vi "Set SysDef Configuration.vi"(8 "error in (no error)":errorcluster, 10 "Configuration":T2={"Name"="", "Description"="", "Protocol"="", "RS232 Config"={"Port"="COM1", "Baud Rate"=9600, "Data Bits"=8, "Parity"=enum."None", "Stop Bits"=10, "Flow Control"=0, "XON"=enum."DC1", "XOFF"=enum."DC3", "End Read on Termination Character"=TRUE, "End Write on Termination Character"=TRUE, "Termination Character"=10}, "MetaData Globals"=[], "Message Groups"=[], "GPIB Config"={"VISA Resource"="GPIB0::2::INSTR", "Enable Termination Character"=TRUE, "Termination Character"=10, "Timeout"=2000, "Append Write Termination Character"=FALSE}, "TCPIP Config"={"IP Address"="localhost", "Port"=0}, "Decimation"=0, "UDP Config"={"Local IP Address"="localhost", "Local Port"=8888, "Target IP Address"="localhost", "Target Port"=8888}} {"GPIB Config"."Termination Character" format="%.0x"; "RS232 Config"."Termination Character" format="%.0x"; "RS232 Config"."Flow Control" items=["None"=0, "XON/XOFF"=1, "RTS/CTS"=2, "DTR/DSR"=4]; "RS232 Config"."Stop Bits" items=["1.0"=10, "1.5"=15, "2.0"=20]; "RS232 Config"."Data Bits" min=5 max=8 step=1; "RS232 Config"."Baud Rate" items=["75"=75, "110"=110, "134"=134, "150"=150, "300"=300, "600"=600, "1200"=1200, "1800"=1800, "2400"=2400, "4800"=4800, "7200"=7200, "9600"=9600, "14400"=14400, "19200"=19200, "28800"=28800, "38400"=38400, "56000"=56000, "57600"=57600, "115200"=115200, "128000"=128000, "230400"=230400, "460800"=460800, "921600"=921600, "1843200"=1843200, "3000000"=3000000]}, 11 "Node Ptr":u64 format="%.0x") -> (0 "error out":errorcluster, 3 "Ref out":T1=18446744073709551615 format="%.0x")   [LabVIEW 2019, in "Instrument Addon System Explorer.lvlib"]
uses:
  Instrument Addon System Explorer.lvlib
  Instrument Custom Device SysDef Configuration V1.0.1.ctl
  Shared/Types/RSXXX Port Settings.ctl
  MetaData Channel Configuration.ctl
  Shared/Types/MetaData Parameters.ctl
  Shared/Types/Protocol Data Type.ctl
  Shared/Types/Metadata Channel Type.ctl
  Shared/Types/Type Cast Type.ctl
  Shared/Types/Endian.ctl
  Types/Channel Properties.ctl
  Message Group Configuration.ctl
  Message Configuration.ctl
  Command Message Configuration.ctl
  Shared/Types/Command Parameters.ctl
  Shared/Types/Linked Channel Cluster.ctl
  Response Message Configuration.ctl
  Shared/Types/Response Parameters.ctl
  Shared/Types/Response Wait Type.ctl
  Data Channel Configuration.ctl
  Shared/Types/Data Parameters.ctl
  Shared/Types/Data Channel Type.ctl
  Shared/Types/Message Parameters.ctl
  Shared/Types/Message Generation Type.ctl
  Shared/Types/Trigger Parameters.ctl
  Shared/Types/VISA Settings.ctl
  Shared/Types/TCPIP Settings.ctl
  Shared/Types/UDP Settings.ctl
  <vilib>/NI VeriStand/Custom Device API/Custom Device Item Ref.ctl
  Shared/Types/FG Control.ctl
  <vilib>/NI VeriStand/Custom Device API/Custom Device Channel.ctl
  <vilib>/NI VeriStand/Custom Device API/Custom Device Channel Type.ctl
  Shared/Constants.vi
  <vilib>/NI VeriStand/Custom Device API/NI VeriStand - Get Item Property.vi
  <vilib>/NI VeriStand/Custom Device API/Get Item Property (U32).vi
  <vilib>/NI VeriStand/Custom Device API/Set Item Property (U32).vi
  <vilib>/NI VeriStand/Custom Device API/Get Item Property (String).vi
  <vilib>/NI VeriStand/Custom Device API/Set Item Property (String).vi
  <vilib>/NI VeriStand/Custom Device API/Get Item Property (Boolean).vi
  <vilib>/NI VeriStand/Custom Device API/Set Item Property (Boolean).vi
  <vilib>/NI VeriStand/Custom Device API/Get Item Property (String Array).vi
  <vilib>/NI VeriStand/Custom Device API/Set Item Property (String Array).vi
  <vilib>/NI VeriStand/Custom Device API/NI VeriStand - Get Item Children.vi
  <vilib>/NI VeriStand/Custom Device API/NI VeriStand - Set Custom Device Channel Value Table.vi
  <vilib>/NI VeriStand/Custom Device API/Get Item Property (Double).vi
  <vilib>/NI VeriStand/Custom Device API/Set Item Property (Double).vi
  <vilib>/NI VeriStand/Custom Device API/Custom Device API.lvlib
  Shared/Instrument Addon Shared.lvlib
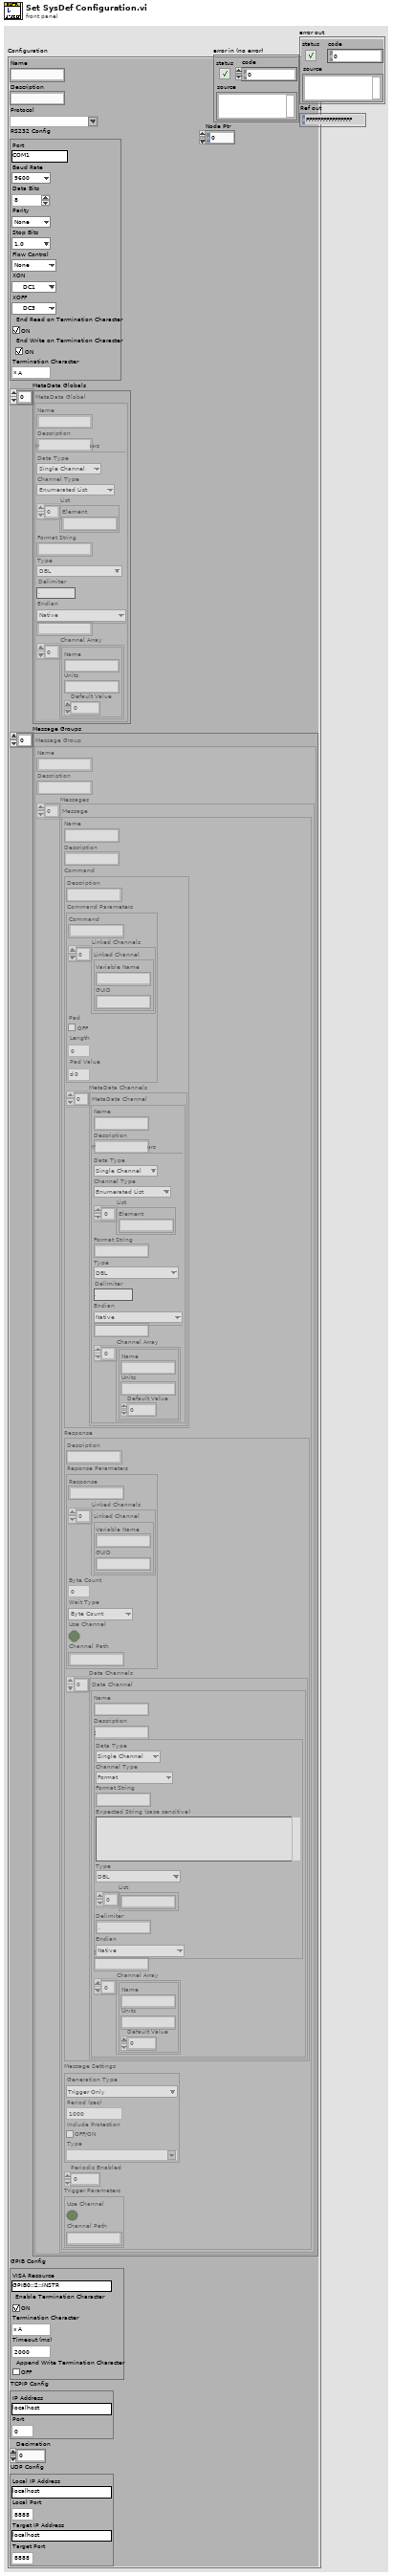
[diagram p1: front panel]
types:
  T1 = typedef "Custom Device API.lvlib/Custom Device Item Ref.ctl" = u64
  T2 = typedef "Instrument Addon System Explorer.lvlib/Instrument Custom Device SysDef Configuration V1.0.1.ctl" = cluster{"Name":string, "Description":string, "Protocol":string, "RS232 Config":T3, "MetaData Globals":T4[], "Message Groups":T11[], "GPIB Config":T25, "TCPIP Config":T26, "Decimation":u32, "UDP Config":T27}
  T3 = typedef "Instrument Addon Shared.lvlib/RSXXX Port Settings.ctl" = cluster{"Port":string, "Baud Rate":u32, "Data Bits":u16, "Parity":enum16{"None", "Odd", "Even", "Mark", "Space"}, "Stop Bits":u16, "Flow Control":u16, "XON":enum16{"NUL", "SOH", "STX", "ETX", "EOT", "ENQ", "ACK", "BEL", "BS", "HT", "LF", "VT", "FF", "CR", "SO", "SI", "DLE", "DC1", "DC2", "DC3", "DC4", "NAK", "SYN", "ETB", "CAN", "EM", "SUB", "ESC", "FS", "GS", "RS", "US", "SP", "!", "\"", "#", "$", "%", "&", "'", "(", ")", "*", "+", ",", "- (-)", ".", "/", "0", "1", "2", "3", "4", "5", "6", "7", "8", "9", ":", ";", "<", "=", ">", "?", "@", "A", "B", "C", "D", "E", "F", "G", "H", "I", "J", "K", "L", "M", "N", "O", "P", "Q", "R", "S", "T", "U", "V", "W", "X", "Y", "Z", "[", "\\", "]", "^", "_", "`", "a", "b", "c", "d", "e", "f", "g", "h", "i", "j", "k", "l", "m", "n", "o", "p", "q", "r", "s", "t", "u", "v", "w", "x", "y", "z", "{", "|", "}", "~"}, "XOFF":enum16{"NUL", "SOH", "STX", "ETX", "EOT", "ENQ", "ACK", "BEL", "BS", "HT", "LF", "VT", "FF", "CR", "SO", "SI", "DLE", "DC1", "DC2", "DC3", "DC4", "NAK", "SYN", "ETB", "CAN", "EM", "SUB", "ESC", "FS", "GS", "RS", "US", "SP", "!", "\"", "#", "$", "%", "&", "'", "(", ")", "*", "+", ",", "- (-)", ".", "/", "0", "1", "2", "3", "4", "5", "6", "7", "8", "9", ":", ";", "<", "=", ">", "?", "@", "A", "B", "C", "D", "E", "F", "G", "H", "I", "J", "K", "L", "M", "N", "O", "P", "Q", "R", "S", "T", "U", "V", "W", "X", "Y", "Z", "[", "\\", "]", "^", "_", "`", "a", "b", "c", "d", "e", "f", "g", "h", "i", "j", "k", "l", "m", "n", "o", "p", "q", "r", "s", "t", "u", "v", "w", "x", "y", "z", "{", "|", "}", "~"}, "End Read on Termination Character":bool, "End Write on Termination Character":bool, "Termination Character":u8}
  T4 = typedef "Instrument Addon System Explorer.lvlib/MetaData Channel Configuration.ctl" = cluster{"Name":string, "Description":string, "MetaData Parameters":T5, "Config GUID":string, "Channel Array":T10[]}
  T5 = typedef "Instrument Addon Shared.lvlib/MetaData Parameters.ctl" = cluster{"Data Type":T6, "Channel Type":T7, "List":string[], "Format String":string, "Type":T8, "Delimiter":string, "Endian":T9}
  T6 = typedef "Instrument Addon Shared.lvlib/Protocol Data Type.ctl" = enum16{"Single Channel", "Array"}
  T7 = typedef "Instrument Addon Shared.lvlib/Metadata Channel Type.ctl" = enum16{"Enumerated List", "Format", "Type Cast"}
  T8 = typedef "Instrument Addon Shared.lvlib/Type Cast Type.ctl" = enum16{"DBL", "SGL", "U64", "U32", "U16", "U8", "I64", "I32", "I16", "I8"}
  T9 = typedef "Instrument Addon Shared.lvlib/Endian.ctl" = enum16{"Native", "Little", "Big"}
  T10 = typedef "Instrument Addon System Explorer.lvlib/Channel Properties.ctl" = cluster{"Name":string, "Units":string, "Default Value":dbl}
  T11 = typedef "Instrument Addon System Explorer.lvlib/Message Group Configuration.ctl" = cluster{"Name":string, "Description":string, "Messages":T12[]}
  T12 = typedef "Instrument Addon System Explorer.lvlib/Message Configuration.ctl" = cluster{"Name":string, "Description":string, "Command":T13, "Response":T16, "Message Settings":T22, "Periodic Enabled":dbl, "Trigger Parameters":T24}
  T13 = typedef "Instrument Addon System Explorer.lvlib/Command Message Configuration.ctl" = cluster{"Description":string, "Command Parameters":T14, "MetaData Channels":T4[]}
  T14 = typedef "Instrument Addon Shared.lvlib/Command Parameters.ctl" = cluster{"Command":string, "Linked Channels":T15[], "Pad":bool, "Length":u32, "Pad Value":u8}
  T15 = typedef "Instrument Addon Shared.lvlib/Linked Channel Cluster.ctl" = cluster{"Variable Name":string, "GUID":string}
  T16 = typedef "Instrument Addon System Explorer.lvlib/Response Message Configuration.ctl" = cluster{"Description":string, "Reponse Parameters":T17, "Data Channels":T19[]}
  T17 = typedef "Instrument Addon Shared.lvlib/Response Parameters.ctl" = cluster{"Response":string, "Linked Channels":T15[], "Type Value":dbl, "Wait Type":T18, "Use Channel":bool, "Channel Path":string}
  T18 = typedef "Instrument Addon Shared.lvlib/Response Wait Type.ctl" = enum16{"Byte Count", "Wait sec"}
  T19 = typedef "Instrument Addon System Explorer.lvlib/Data Channel Configuration.ctl" = cluster{"Name":string, "Description":string, "Data Parameters":T20, "Config GUID":string, "Channel Array":T10[]}
  T20 = typedef "Instrument Addon Shared.lvlib/Data Parameters.ctl" = cluster{"Data Type":T6, "Channel Type":T21, "Format String":string, "Expected String":string, "Type":T8, "List":string[], "Delimiter":string, "Endian":T9}
  T21 = typedef "Instrument Addon Shared.lvlib/Data Channel Type.ctl" = enum16{"Format", "Comparison", "Type Cast", "Enumerated List"}
  T22 = typedef "Instrument Addon Shared.lvlib/Message Parameters.ctl" = cluster{"Generation Type":T23, "Period":dbl, "Include Protection":bool, "Type":string}
  T23 = typedef "Instrument Addon Shared.lvlib/Message Generation Type.ctl" = enum16{"Trigger Only", "Periodic & Trigger", "Value Change & Trigger"}
  T24 = typedef "Instrument Addon Shared.lvlib/Trigger Parameters.ctl" = cluster{"Use Channel":bool, "Channel Path":string}
  T25 = typedef "Instrument Addon Shared.lvlib/VISA Settings.ctl" = cluster{"VISA Resource":string, "Enable Termination Character":bool, "Termination Character":u8, "Timeout":u32, "Append Write Termination Character":bool}
  T26 = typedef "Instrument Addon Shared.lvlib/TCPIP Settings.ctl" = cluster{"IP Address":string, "Port":u16}
  T27 = typedef "Instrument Addon Shared.lvlib/UDP Settings.ctl" = cluster{"Local IP Address":string, "Local Port":u16, "Target IP Address":string, "Target Port":u16}
  T28 = typedef "Instrument Addon Shared.lvlib/FG Control.ctl" = enum16{"Get", "Set"}
  T29 = typedef "Custom Device API.lvlib/Custom Device Channel.ctl" = cluster{"Type":T30, "Units":string, "Default Value":dbl, "Faultable":bool, "Scalable":bool}
  T30 = typedef "Custom Device API.lvlib/Custom Device Channel Type.ctl" = enum16{"Input", "Output"}
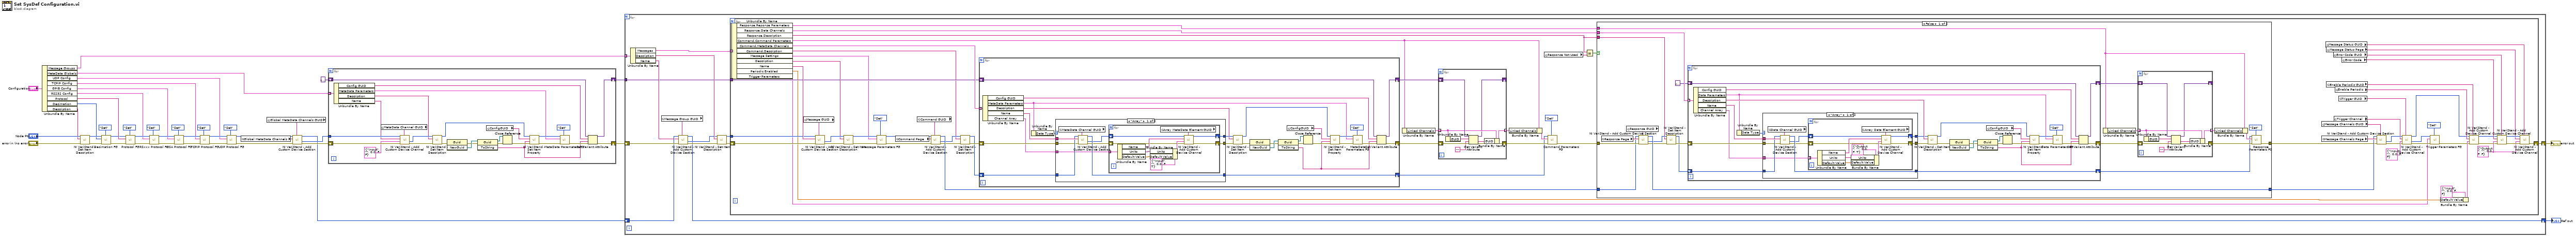
[diagram p0: block diagram]
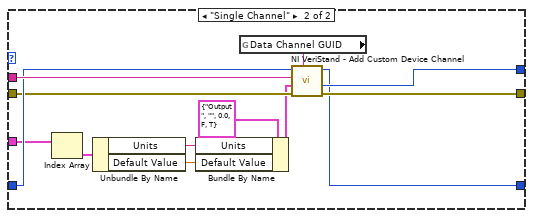
[diagram p2: hidden frame]
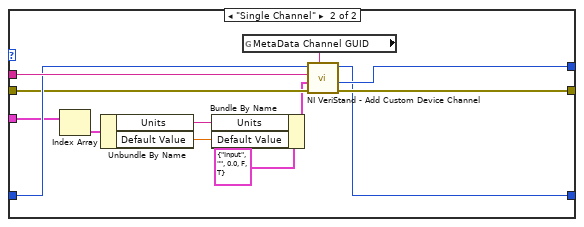
[diagram p4: hidden frame]
diagram:
  n1 = Unbundle By Name("Configuration") -> ("Message Groups"=w24:T11[], "MetaData Globals"=w29:T4[], "UDP Config"=w1:T27, "TCPIP Config"=w13:T26, "GPIB Config"=w16:T25, "RS232 Config"=w32:T3, "Protocol"=w33:string, "Decimation"=w7:u32, "Description"=w34:string)
  n2 = call <vilib>:"NI VeriStand - Set Item Description.vi"("error in (no error)"="error in (no error)", "Description"=w34, "Item Ref in"="Node Ptr") -> ("error out"=w10:errorcluster, "Item Ref out"=w35:T1)  [unwired: 6 in, 1 out]
  n3 = call "Decimation FG.vi"("Action"=FG_Control."Set", "error in (no error)"=w10, "Decimation"=w7, "Device Item Ref in"=w35) -> ("error out"=w9:errorcluster, "Item Ref out"=w11:T1)  [unwired: 5 in, 1 out]
  n4 = call "Protocol FG.vi"("Action"=FG_Control."Set", "error in (no error)"=w9, "Protocol"=w33, "Device Item Ref in"=w11) -> ("error out"=w41:errorcluster, "Item Ref out"=w40:T1)  [unwired: 5 in, 1 out]
  n5 = call "RSxxx Protocol FG.vi"("Action"=FG_Control."Set", "error in (no error)"=w41, "Serial Config"=w32, "Device Item Ref in"=w40) -> ("error out"=w19:errorcluster, "Item Ref out"=w17:T1)  [unwired: 5 in, 1 out]
  n6 = call "VISA Protocol FG.vi"("Action"=FG_Control."Set", "error in (no error)"=w19, "VISA Config"=w16, "Device Item Ref in"=w17) -> ("error out"=w18:errorcluster, "Item Ref out"=w14:T1)  [unwired: 5 in, 1 out]
  n7 = call "TCPIP Protocol FG.vi"("Action"=FG_Control."Set", "error in (no error)"=w18, "TCP/IP Config"=w13, "Device Item Ref in"=w14) -> ("error out"=w6:errorcluster, "Item Ref out"=w4:T1)  [unwired: 5 in, 1 out]
  n8 = call "UDP Protocol FG.vi"("Action"=FG_Control."Set", "error in (no error)"=w6, "UDP Config"=w1, "Device Item Ref in"=w4) -> ("error out"=w5:errorcluster, "Item Ref out"=w3:T1)  [unwired: 5 in, 1 out]
  n9 = global read "Constants.vi" "Global MetaData Channels"() -> (w30:string)
  n10 = global read "Constants.vi" "Global MetaData Channels GUID"() -> (w31:string)
  n11 = call <vilib>:"NI VeriStand - Add Custom Device Section.vi"("GUID (Default Section)"=w31, "error in (no error)"=w5, "Section Name"=w30, "Parent Ref in"=w3) -> ("error out"=w28:errorcluster, "Section Ptr"=w27:T1, "Parent Ref out"=w23:T1)  [unwired: 4 in, 1 out]
  n12 = for {
    tunnel: w29 -> [w69] mode=indexing
    tunnel: w27 -> [w61]
    shift-right: [w45] -> w22
    shift-left: variant ("variant") -> [w46]
    shift-right: [w44] -> w25
    shift-left: w28 -> [w62]
    n13 = Unbundle By Name(w69) -> ("Config GUID"=w48:string, "MetaData Parameters"=w50:T5, "Description"=w54:string, "Name"=w59:string)
    n14 = global read "Constants.vi" "MetaData Channel GUID"() -> (w60:string)
    n15 = call <vilib>:"NI VeriStand - Add Custom Device Channel.vi"("GUID (Default Channel)"=w60, "error in (no error)"=w62, "Channel"=T29 {"Type"=enum."Input", "Units"="", "Default Value"=0.0, "Faultable"=FALSE, "Scalable"=FALSE}, "Channel Name"=w59, "Parent Ref in"=w61) -> ("error out"=w58:errorcluster, "Channel Ref"=w56:T1)  [unwired: 3 in, 2 out]
    n16 = call <vilib>:"NI VeriStand - Set Item Description.vi"("error in (no error)"=w58, "Description"=w54, "Item Ref in"=w56) -> ("error out"=w57:errorcluster, "Item Ref out"=w55:T1)  [unwired: 6 in, 1 out]
    n17 = invoke class="Guid" method="NewGuid"(error in=w57) -> (error out=w65:errorcluster, "NewGuid"=w66:refnum<k24>)  [unwired: 2 in, 1 out]
    n18 = invoke class="Guid" method="ToString"(reference=w66, error in=w65) -> (reference out=w67:refnum<k24>, error out=w64:errorcluster, "ToString"=w47:string)  [unwired: 1 in]
    n19 = global read "Constants.vi" "ConfigGUID"() -> (w68:string)
    n20 = Close Reference(reference=w67, error in (no error)=w64) -> (error out=w63:errorcluster)
    n21 = call-poly <vilib>:"NI VeriStand - Set Item Property.vi"("error in (no error)"=w63, "Value"=w47, "Property Name"=w68, "Item Ref in"=w55) -> ("error out"=w53:errorcluster, "Item Ref out"=w52:T1)  [unwired: 5 in, 1 out]
    n22 = call "MetaData Parameters FG.vi"("Action"=FG_Control."Set", "error in (no error)"=w53, "MetaData Parameters"=w50, "Item Ref in"=w52) -> ("error out"=w49:errorcluster)  [unwired: 5 in, 2 out]
    n23 = Set Variant Attribute(Variant=w46, name=w48, value=w47, error in=w49) -> (Variant out=w45:variant, error out=w44:errorcluster)  [unwired: 1 out]
  }
  n24 = for {
    shift-right: [w72] -> w21
    shift-left: w25 -> [w82]
    tunnel: w24 -> [w81] mode=indexing
    tunnel: w22 -> [w73]
    shift-right: [w70] -> w20
    shift-left: w23 -> [w79]
    n25 = Unbundle By Name(w81) -> ("Messages"=w76:T12[], "Description"=w77:string, "Name"=w78:string)
    n26 = global read "Constants.vi" "Message Group GUID"() -> (w83:string)
    n27 = call <vilib>:"NI VeriStand - Add Custom Device Section.vi"("GUID (Default Section)"=w83, "error in (no error)"=w82, "Section Name"=w78, "Parent Ref in"=w79) -> ("error out"=w80:errorcluster, "Section Ptr"=w71:T1, "Parent Ref out"=w70:T1)  [unwired: 4 in, 1 out]
    n28 = call <vilib>:"NI VeriStand - Set Item Description.vi"("error in (no error)"=w80, "Description"=w77, "Item Ref in"=w71) -> ("error out"=w75:errorcluster, "Item Ref out"=w74:T1)  [unwired: 6 in, 1 out]
    n29 = for {
      tunnel: w76 -> [w152] mode=indexing
      shift-right: [w110] -> w72
      shift-left: w75 -> [w132]
      tunnel: w74 -> [w133]
      tunnel: w73 -> [w113]
      w137 = T29 {"Type"=enum."Output", "Units"="", "Default Value"=0.0, "Faultable"=FALSE, "Scalable"=FALSE} ("Channel")
      n30 = Unbundle By Name(w152) -> ("Response.Reponse Parameters"=w111:T17, "Response.Data Channels"=w114:T19[], "Response.Description"=w92:string, "Command.Command Parameters"=w121:T14, "Command.MetaData Channels"=w126:T4[], "Command.Description"=w105:string, "Message Settings"=w98:T22, "Description"=w128:string, "Name"=w134:string, "Periodic Enabled"=w90:dbl, "Trigger Parameters"=w84:T24)
      n31 = global read "Constants.vi" "Message GUID"() -> (w150:string)
      n32 = call <vilib>:"NI VeriStand - Add Custom Device Section.vi"("GUID (Default Section)"=w150, "error in (no error)"=w132, "Section Name"=w134, "Parent Ref in"=w133) -> ("error out"=w131:errorcluster, "Section Ptr"=w129:T1)  [unwired: 4 in, 2 out]
      n33 = call <vilib>:"NI VeriStand - Set Item Description.vi"("error in (no error)"=w131, "Description"=w128, "Item Ref in"=w129) -> ("error out"=w130:errorcluster, "Item Ref out"=w103:T1)  [unwired: 6 in, 1 out]
      n34 = call "Message Parameters FG.vi"("Action"=FG_Control."Set", "error in (no error)"=w130, "Message Settings"=w98, "Item Ref in"=w103) -> ("error out"=w104:errorcluster, "Item Ref out"=w102:T1)  [unwired: 5 in, 1 out]
      n35 = global read "Constants.vi" "Command Page"() -> (w140:string)
      n36 = global read "Constants.vi" "Command GUID"() -> (w141:string)
      n37 = call <vilib>:"NI VeriStand - Add Custom Device Section.vi"("GUID (Default Section)"=w141, "error in (no error)"=w104, "Section Name"=w140, "Parent Ref in"=w102) -> ("error out"=w109:errorcluster, "Section Ptr"=w107:T1, "Parent Ref out"=w115:T1)  [unwired: 4 in, 1 out]
      n38 = call <vilib>:"NI VeriStand - Set Item Description.vi"("error in (no error)"=w109, "Description"=w105, "Item Ref in"=w107) -> ("error out"=w108:errorcluster, "Item Ref out"=w106:T1)  [unwired: 6 in, 1 out]
      n39 = for {
        tunnel: w126 -> [w263] mode=indexing
        shift-right: [w262] -> w125
        shift-left: w108 -> [w264]
        shift-right: [w266] -> w123
        shift-left: w113 -> [w267]
        shift-right: [w261] -> w116
        shift-left: w106 -> [w265]
        n40 = Unbundle By Name(w263) -> ("Config GUID"=w268:string, "MetaData Parameters"=w259:T5, "Description"=w273:string, "Name"=w278:string, "Channel Array"=w257:T10[])
        n41 = Unbundle By Name(w259) -> ("Data Type"=w258:T6)
        n42 = case shown="\"Array\"" w258 {
          tunnel: w278 -> [w293 w317]
          tunnel: [w286 w316] -> w277
          tunnel: [w285 w315] -> w275
          tunnel: w265 -> [w292 w314]
          tunnel: w264 -> [w291 w313]
          tunnel: [w290 w312] -> w261
          tunnel: w257 -> [w287 w310]
          frame "Array" {
            n43 = global read "Constants.vi" "MetaData Channel GUID"() -> (w294:string)
            n44 = call <vilib>:"NI VeriStand - Add Custom Device Section.vi"("GUID (Default Section)"=w294, "error in (no error)"=w291, "Section Name"=w293, "Parent Ref in"=w292) -> ("error out"=w288:errorcluster, "Section Ptr"=w289:T1, "Parent Ref out"=w290:T1)  [unwired: 4 in, 1 out]
            n45 = for {
              shift-right: [w298] -> w285
              shift-left: w289 -> [w305]
              shift-right: [w297] -> w286
              shift-left: w288 -> [w296]
              tunnel: w287 -> [w304] mode=indexing
              n46 = Unbundle By Name(w304) -> ("Name"=w303:string, "Units"=w302:string, "Default Value"=w301:dbl)
              n47 = Bundle By Name(cluster=T29 {"Type"=enum."Input", "Units"="", "Default Value"=0.0, "Faultable"=FALSE, "Scalable"=TRUE} ("Channel"), "Units"=w302, "Default Value"=w301) -> (w300:T29)
              n48 = global read "Constants.vi" "Array MetaData Element GUID"() -> (w299:string)
              n49 = call <vilib>:"NI VeriStand - Add Custom Device Channel.vi"("GUID (Default Channel)"=w299, "error in (no error)"=w296, "Channel"=w300, "Channel Name"=w303, "Parent Ref in"=w305) -> ("error out"=w297:errorcluster, "Parent Ref out"=w298:T1)  [unwired: 3 in, 2 out]
            }
          }
          frame "Single Channel" {
            n50 = Index Array(array=w310) -> (element=w309:T10)  [unwired: 1 in]
            n51 = Unbundle By Name(w309) -> ("Units"=w308:string, "Default Value"=w307:dbl)
            n52 = Bundle By Name(cluster=T29 {"Type"=enum."Input", "Units"="", "Default Value"=0.0, "Faultable"=FALSE, "Scalable"=TRUE} ("Channel"), "Units"=w308, "Default Value"=w307) -> (w311:T29)
            n53 = global read "Constants.vi" "MetaData Channel GUID"() -> (w318:string)
            n54 = call <vilib>:"NI VeriStand - Add Custom Device Channel.vi"("GUID (Default Channel)"=w318, "error in (no error)"=w313, "Channel"=w311, "Channel Name"=w317, "Parent Ref in"=w314) -> ("error out"=w316:errorcluster, "Channel Ref"=w315:T1, "Parent Ref out"=w312:T1)  [unwired: 3 in, 1 out]
          }
        }
        n55 = call <vilib>:"NI VeriStand - Set Item Description.vi"("error in (no error)"=w277, "Description"=w273, "Item Ref in"=w275) -> ("error out"=w276:errorcluster, "Item Ref out"=w274:T1)  [unwired: 6 in, 1 out]
        n56 = invoke class="Guid" method="NewGuid"(error in=w276) -> (error out=w281:errorcluster, "NewGuid"=w282:refnum<k24>)  [unwired: 2 in, 1 out]
        n57 = invoke class="Guid" method="ToString"(reference=w282, error in=w281) -> (reference out=w283:refnum<k24>, error out=w280:errorcluster, "ToString"=w260:string)  [unwired: 1 in]
        n58 = global read "Constants.vi" "ConfigGUID"() -> (w284:string)
        n59 = Close Reference(reference=w283, error in (no error)=w280) -> (error out=w279:errorcluster)
        n60 = call-poly <vilib>:"NI VeriStand - Set Item Property.vi"("error in (no error)"=w279, "Value"=w260, "Property Name"=w284, "Item Ref in"=w274) -> ("error out"=w272:errorcluster, "Item Ref out"=w271:T1)  [unwired: 5 in, 1 out]
        n61 = call "MetaData Parameters FG.vi"("Action"=FG_Control."Set", "error in (no error)"=w272, "MetaData Parameters"=w259, "Item Ref in"=w271) -> ("error out"=w269:errorcluster)  [unwired: 5 in, 2 out]
        n62 = Set Variant Attribute(Variant=w267, name=w268, value=w260, error in=w269) -> (Variant out=w266:variant, error out=w262:errorcluster)  [unwired: 1 out]
      }
      n63 = Unbundle By Name(w121) -> ("Linked Channels"=w124:T15[])
      n64 = for {
        shift-right: [w249] -> w119
        shift-left: w125 -> [w256]
        tunnel: w124 -> [w252] mode=indexing
        shift-right: [w248] -> _
        shift-left: w123 -> [w255]
        tunnel: [w250] -> w122 mode=indexing
        n65 = Unbundle By Name(w252) -> ("GUID"=w254:string)
        n66 = Get Variant Attribute(Variant=w255, name=w254, default value (empty Variant)="", error in=w256) -> (duplicate Variant=w248:variant, value=w251:string, error out=w249:errorcluster)  [unwired: 1 out]
        n67 = Bundle By Name(cluster=w252, "GUID"=w251) -> (w250:T15)
      }
      n68 = Bundle By Name(cluster=w121, "Linked Channels"=w122) -> (w120:T14)
      n69 = global read "Constants.vi" "Response Not Used"() -> (w93:string)
      n70 = call "Command Parameters FG.vi"("Action"=FG_Control."Set", "error in (no error)"=w119, "Command Parameters"=w120, "Item Ref in"=w116) -> ("error out"=w118:errorcluster)  [unwired: 5 in, 2 out]
      n71 = Equal?(x=w92, y=w93) -> (x = y?=w91:bool)
      n72 = case shown="False" w91 {
        tunnel: w118 -> [w172 w246]
        tunnel: [w171 w247] -> w117
        tunnel: w115 -> [w170 w247]
        tunnel: w114 -> [w169 _]
        tunnel: [w163 w246] -> w112
        tunnel: w111 -> [w162 _]
        tunnel: w92 -> [w154 _]
        frame False {
          n73 = global read "Constants.vi" "Response Page"() -> (w174:string)
          n74 = global read "Constants.vi" "Response GUID"() -> (w173:string)
          n75 = call <vilib>:"NI VeriStand - Add Custom Device Section.vi"("GUID (Default Section)"=w173, "error in (no error)"=w172, "Section Name"=w174, "Parent Ref in"=w170) -> ("error out"=w158:errorcluster, "Section Ptr"=w156:T1, "Parent Ref out"=w171:T1)  [unwired: 4 in, 1 out]
          n76 = call <vilib>:"NI VeriStand - Set Item Description.vi"("error in (no error)"=w158, "Description"=w154, "Item Ref in"=w156) -> ("error out"=w157:errorcluster, "Item Ref out"=w155:T1)  [unwired: 6 in, 1 out]
          n77 = for {
            tunnel: w169 -> [w194] mode=indexing
            shift-right: [w193] -> w167
            shift-left: w157 -> [w190]
            shift-right: [w195] -> w166
            shift-left: variant ("variant") -> [w196]
            shift-right: [w191] -> w159
            shift-left: w155 -> [w192]
            n78 = Unbundle By Name(w194) -> ("Config GUID"=w198:string, "Data Parameters"=w186:T20, "Description"=w203:string, "Name"=w189:string, "Channel Array"=w184:T10[])
            n79 = Unbundle By Name(w186) -> ("Data Type"=w185:T6)
            n80 = case shown="\"Array\"" w185 {
              tunnel: w189 -> [w221 w245]
              tunnel: [w214 w244] -> w187
              tunnel: [w213 w243] -> w188
              tunnel: w192 -> [w220 w242]
              tunnel: w190 -> [w219 w241]
              tunnel: [w218 w240] -> w191
              tunnel: w184 -> [w215 w238]
              frame "Array" {
                n81 = global read "Constants.vi" "Data Channel GUID"() -> (w212:string)
                n82 = call <vilib>:"NI VeriStand - Add Custom Device Section.vi"("GUID (Default Section)"=w212, "error in (no error)"=w219, "Section Name"=w221, "Parent Ref in"=w220) -> ("error out"=w216:errorcluster, "Section Ptr"=w217:T1, "Parent Ref out"=w218:T1)  [unwired: 4 in, 1 out]
                n83 = for {
                  shift-right: [w225] -> w213
                  shift-left: w217 -> [w232]
                  shift-right: [w224] -> w214
                  shift-left: w216 -> [w223]
                  tunnel: w215 -> [w231] mode=indexing
                  n84 = Unbundle By Name(w231) -> ("Name"=w230:string, "Units"=w229:string, "Default Value"=w228:dbl)
                  n85 = Bundle By Name(cluster=T29 {"Type"=enum."Output", "Units"="", "Default Value"=0.0, "Faultable"=FALSE, "Scalable"=TRUE} ("Channel"), "Units"=w229, "Default Value"=w228) -> (w227:T29)
                  n86 = global read "Constants.vi" "Array Data Element GUID"() -> (w226:string)
                  n87 = call <vilib>:"NI VeriStand - Add Custom Device Channel.vi"("GUID (Default Channel)"=w226, "error in (no error)"=w223, "Channel"=w227, "Channel Name"=w230, "Parent Ref in"=w232) -> ("error out"=w224:errorcluster, "Parent Ref out"=w225:T1)  [unwired: 3 in, 2 out]
                }
              }
              frame "Single Channel" {
                n88 = Index Array(array=w238) -> (element=w237:T10)  [unwired: 1 in]
                n89 = Unbundle By Name(w237) -> ("Units"=w236:string, "Default Value"=w235:dbl)
                n90 = Bundle By Name(cluster=T29 {"Type"=enum."Output", "Units"="", "Default Value"=0.0, "Faultable"=FALSE, "Scalable"=TRUE} ("Channel"), "Units"=w236, "Default Value"=w235) -> (w239:T29)
                n91 = global read "Constants.vi" "Data Channel GUID"() -> (w234:string)
                n92 = call <vilib>:"NI VeriStand - Add Custom Device Channel.vi"("GUID (Default Channel)"=w234, "error in (no error)"=w241, "Channel"=w239, "Channel Name"=w245, "Parent Ref in"=w242) -> ("error out"=w244:errorcluster, "Channel Ref"=w243:T1, "Parent Ref out"=w240:T1)  [unwired: 3 in, 1 out]
              }
            }
            n93 = call <vilib>:"NI VeriStand - Set Item Description.vi"("error in (no error)"=w187, "Description"=w203, "Item Ref in"=w188) -> ("error out"=w205:errorcluster, "Item Ref out"=w204:T1)  [unwired: 6 in, 1 out]
            n94 = invoke class="Guid" method="NewGuid"(error in=w205) -> (error out=w208:errorcluster, "NewGuid"=w209:refnum<k24>)  [unwired: 2 in, 1 out]
            n95 = invoke class="Guid" method="ToString"(reference=w209, error in=w208) -> (reference out=w210:refnum<k24>, error out=w207:errorcluster, "ToString"=w197:string)  [unwired: 1 in]
            n96 = global read "Constants.vi" "ConfigGUID"() -> (w211:string)
            n97 = Close Reference(reference=w210, error in (no error)=w207) -> (error out=w206:errorcluster)
            n98 = call-poly <vilib>:"NI VeriStand - Set Item Property.vi"("error in (no error)"=w206, "Value"=w197, "Property Name"=w211, "Item Ref in"=w204) -> ("error out"=w202:errorcluster, "Item Ref out"=w201:T1)  [unwired: 5 in, 1 out]
            n99 = call "Data Parameters FG.vi"("Action"=FG_Control."Set", "error in (no error)"=w202, "Data Parameters"=w186, "Item Ref in"=w201) -> ("error out"=w199:errorcluster)  [unwired: 5 in, 2 out]
            n100 = Set Variant Attribute(Variant=w196, name=w198, value=w197, error in=w199) -> (Variant out=w195:variant, error out=w193:errorcluster)  [unwired: 1 out]
          }
          n101 = Unbundle By Name(w162) -> ("Linked Channels"=w165:T15[])
          n102 = for {
            shift-right: [w176] -> w164
            shift-left: w167 -> [w183]
            tunnel: w165 -> [w179] mode=indexing
            shift-right: [w175] -> _
            shift-left: w166 -> [w182]
            tunnel: [w177] -> w161 mode=indexing
            n103 = Unbundle By Name(w179) -> ("GUID"=w181:string)
            n104 = Get Variant Attribute(Variant=w182, name=w181, default value (empty Variant)="", error in=w183) -> (duplicate Variant=w175:variant, value=w178:string, error out=w176:errorcluster)  [unwired: 1 out]
            n105 = Bundle By Name(cluster=w179, "GUID"=w178) -> (w177:T15)
          }
          n106 = Bundle By Name(cluster=w162, "Linked Channels"=w161) -> (w160:T17)
          n107 = call "Response Parameters FG.vi"("Action"=FG_Control."Set", "error in (no error)"=w164, "Reponse Parameters"=w160, "Item Ref in"=w159) -> ("error out"=w163:errorcluster)  [unwired: 5 in, 2 out]
        }
        frame True {
        }
      }
      n108 = global read "Constants.vi" "Message Channels GUID"() -> (w148:string)
      n109 = global read "Constants.vi" "Message Channels Page"() -> (w149:string)
      n110 = global read "Constants.vi" "Message Status GUID"() -> (w136:string)
      n111 = global read "Constants.vi" "Message Status Page"() -> (w135:string)
      n112 = global read "Constants.vi" "Enable Periodic GUID"() -> (w97:string)
      n113 = global read "Constants.vi" "Error Code GUID"() -> (w143:string)
      n114 = global read "Constants.vi" "Trigger Channel"() -> (w144:string)
      n115 = global read "Constants.vi" "Enable Periodic"() -> (w96:string)
      n116 = global read "Constants.vi" "Trigger GUID"() -> (w145:string)
      n117 = global read "Constants.vi" "Error Code"() -> (w142:string)
      n118 = call <vilib>:"NI VeriStand - Add Custom Device Section.vi"("GUID (Default Section)"=w148, "error in (no error)"=w112, "Section Name"=w149, "Parent Ref in"=w117) -> ("error out"=w147:errorcluster, "Section Ptr"=w146:T1)  [unwired: 4 in, 2 out]
      n119 = call <vilib>:"NI VeriStand - Add Custom Device Channel.vi"("GUID (Default Channel)"=w145, "error in (no error)"=w147, "Channel"=T29 {"Type"=enum."Input", "Units"="", "Default Value"=0.0, "Faultable"=FALSE, "Scalable"=FALSE}, "Channel Name"=w144, "Parent Ref in"=w146) -> ("error out"=w88:errorcluster, "Channel Ref"=w89:T1, "Parent Ref out"=w85:T1)  [unwired: 3 in, 1 out]
      n120 = call "Trigger Parameters FG.vi"("Action"=FG_Control."Set", "error in (no error)"=w88, "Trigger Parameters"=w84, "Item Ref in"=w89) -> ("error out"=w87:errorcluster)  [unwired: 5 in, 2 out]
      n121 = Bundle By Name(cluster=T29 {"Type"=enum."Input", "Units"="", "Default Value"=0.0, "Faultable"=FALSE, "Scalable"=FALSE} ("Channel"), "Default Value"=w90) -> (w94:T29)
      n122 = call <vilib>:"NI VeriStand - Add Custom Device Channel.vi"("GUID (Default Channel)"=w97, "error in (no error)"=w87, "Channel"=w94, "Channel Name"=w96, "Parent Ref in"=w85) -> ("error out"=w100:errorcluster, "Parent Ref out"=w99:T1)  [unwired: 3 in, 2 out]
      n123 = call <vilib>:"NI VeriStand - Add Custom Device Channel.vi"("GUID (Default Channel)"=w143, "error in (no error)"=w100, "Channel"=w137, "Channel Name"=w142, "Parent Ref in"=w99) -> ("error out"=w139:errorcluster, "Parent Ref out"=w138:T1)  [unwired: 3 in, 2 out]
      n124 = call <vilib>:"NI VeriStand - Add Custom Device Channel.vi"("GUID (Default Channel)"=w136, "error in (no error)"=w139, "Channel"=w137, "Channel Name"=w135, "Parent Ref in"=w138) -> ("error out"=w110:errorcluster)  [unwired: 3 in, 3 out]
    }
  }
  "error out" <- w21
  "Ref out" <- w20
